vi "DigitalOutput-Drive.vi"(7 "duration (-1 = cont.)":i32=-1, 8 "error in":errorcluster, 9 "data":bool[](array[boolean]), 10 "line+TS":refnum<k21>, 11 "line only":refnum<k21>) -> (0 "error out":errorcluster)   [LabVIEW 2015]
doc: "Drives a DAQmx task [line only] to the level specified in the 1D Boolean array [data]. \n\nIf [duration] is nonnegative, then it will drive the task to ~[data] after the specified duration (ms). This is done using an asynchronous call to DigitalOutput-ScheduledDAQmxWrite.vi\n\nIf [line+TS] is a valid task (where a single timestamp line has been appended to the original task), then it will also pulse the timestamp line. The rising edge of this pulse is synchronized with the start of driving the line.\n\nIf [line+TS] is a valid task and [duration] is negative, then the [line only] task will never be driven. You can use this (with [data] as an empty array) to produce timestamp pulses.\n\nTiming warnings: The timestamp pulse is a 100-200 microsecond high pulse."
uses:
  <vilib>/DAQmx/write.llb/DAQmx Write (Digital 1D Bool NChan 1Samp 1Line).vi
  <vilib>/DAQmx/miscellaneous.llb/DAQmx Fill In Error Info.vi
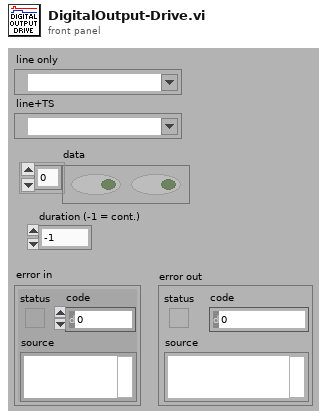
[diagram p1: front panel]
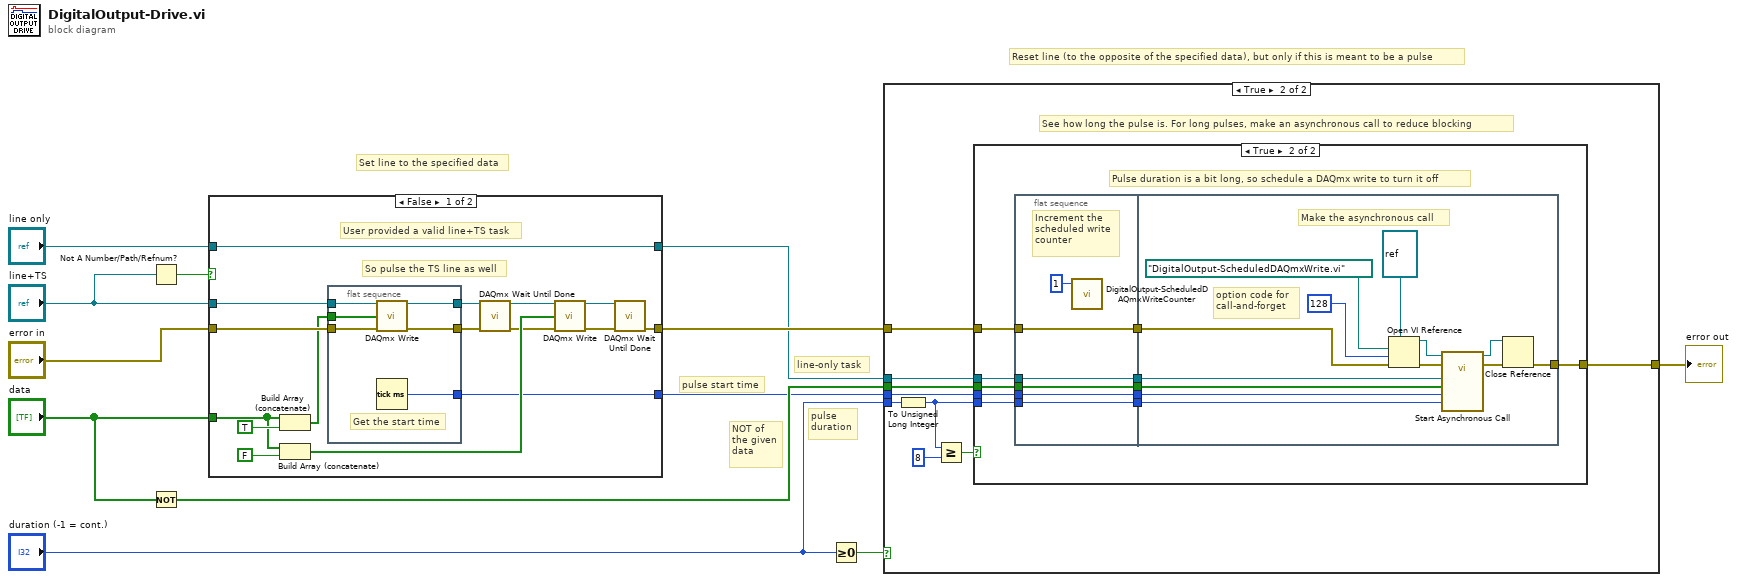
[diagram p0: block diagram]
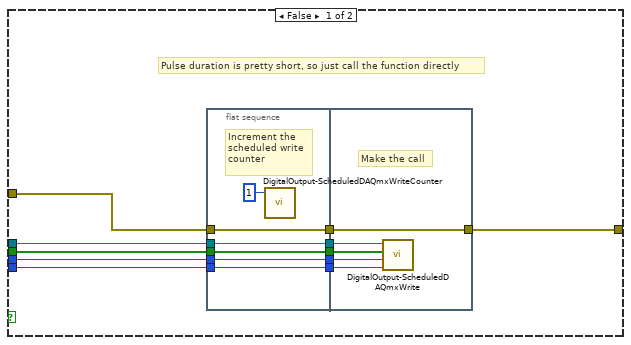
[diagram p3: hidden frame]
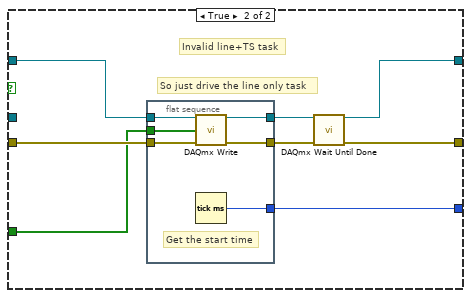
[diagram p4: hidden frame]
diagram:
  # "NOT of \nthe given\ndata"
  # "pulse\nduration"
  # "pulse start time"
  # "line-only task"
  # "Reset line (to the opposite of the specified data), but only if this is meant to be a pulse"
  # "Set line to the specified data"
  n1 = Not A Number/Path/Refnum?(number/path/refnum="line+TS") -> (NaN/Path/Refnum?=w12:bool)
  n2 = Not(x="data") -> (.not. x?=w6:bool[])
  n3 = case shown="False" w12 {
    tunnel: "line only" -> [w25 w42]
    tunnel: "line+TS" -> [w24 _]
    tunnel: "data" -> [w26 w36]
    tunnel: [w25 w39] -> w5
    tunnel: "error in" -> [w23 w37]
    tunnel: [w18 w38] -> w7
    tunnel: [w17 w35] -> w4
    frame False {
      # "User provided a valid line+TS task"
      # "So pulse the TS line as well"
      n4 = Build Array (concatenate)(w26, TRUE) -> (w22:bool[])
      n5 = Build Array (concatenate)(w26, FALSE) -> (w21:bool[])
      n6 = flat-sequence {
        tunnel: w24 -> [w34]
        tunnel: w23 -> [w33]
        tunnel: w22 -> [w32]
        tunnel: [w31] -> w16
        tunnel: [w30] -> w15
        tunnel: [w29] -> w17
        frame #0 {
          # "Get the start time"
          n7 = call-poly <vilib>:"DAQmx Write.vi"("task/channels in"=w34, "data"=w32, "error in"=w33) -> ("task out"=w31:refnum<k21>, "error out"=w30:errorcluster)  [unwired: 10 in, 1 out]
          n8 = Tick Count (ms)() -> (millisecond timer value=w29:u32)
        }
      }
      n9 = call <vilib>:"DAQmx Wait Until Done.vi"("task/channels in"=w16, "error in"=w15) -> ("task out"=w14:refnum<k21>, "error out"=w13:errorcluster)  [unwired: 12 in]
      n10 = call-poly <vilib>:"DAQmx Write.vi"("task/channels in"=w14, "data"=w21, "error in"=w13) -> ("task out"=w20:refnum<k21>, "error out"=w19:errorcluster)  [unwired: 10 in, 1 out]
      n11 = call <vilib>:"DAQmx Wait Until Done.vi"("task/channels in"=w20, "error in"=w19) -> ("error out"=w18:errorcluster)  [unwired: 12 in, 1 out]
    }
    frame True {
      # "So just drive the line only task"
      # "Invalid line+TS task"
      n12 = flat-sequence {
        tunnel: w42 -> [w48]
        tunnel: [w47] -> w41
        tunnel: [w46] -> w40
        tunnel: w37 -> [w45]
        tunnel: w36 -> [w44]
        tunnel: [w43] -> w35
        frame #0 {
          # "Get the start time"
          n13 = call-poly <vilib>:"DAQmx Write.vi"("task/channels in"=w48, "data"=w44, "error in"=w45) -> ("task out"=w47:refnum<k21>, "error out"=w46:errorcluster)  [unwired: 10 in, 1 out]
          n14 = Tick Count (ms)() -> (millisecond timer value=w43:u32)
        }
      }
      n15 = call <vilib>:"DAQmx Wait Until Done.vi"("task/channels in"=w41, "error in"=w40) -> ("task out"=w39:refnum<k21>, "error out"=w38:errorcluster)  [unwired: 12 in]
    }
  }
  n16 = Greater Or Equal To 0?(x="duration (-1 = cont.)") -> (x >= 0?=w2:bool)
  n17 = case shown="True" w2 {
    tunnel: w7 -> [w49 w58]
    tunnel: w6 -> [_ w57]
    tunnel: w5 -> [_ w56]
    tunnel: w4 -> [_ w55]
    tunnel: "duration (-1 = cont.)" -> [_ w54]
    tunnel: [w49 w53] -> w1
    frame False {
      # "Pulse duration negative, so this is supposed to be a\ncontinuous drive. So leave it as it is. Do nothing."
    }
    frame True {
      # "See how long the pulse is. For long pulses, make an asynchronous call to reduce blocking"
      n18 = To Unsigned Long Integer(number=w54) -> (unsigned 32bit integer=w52:u32)
      n19 = Greater Or Equal?(x=w52, y=u32 8) -> (x >= y?=w50:bool)
      n20 = case shown="True" w50 {
        tunnel: w58 -> [w64 w86]
        tunnel: w57 -> [w62 w85]
        tunnel: w56 -> [w63 w84]
        tunnel: w55 -> [w61 w83]
        tunnel: [w59 w82] -> w53
        tunnel: w52 -> [w60 w81]
        frame False {
          # "Pulse duration is pretty short, so just call the function directly"
          n21 = flat-sequence {
            tunnel: w60 -> [w71]
            tunnel: w61 -> [w72]
            tunnel: w63 -> [w73]
            tunnel: w62 -> [w74]
            tunnel: w64 -> [w75]
            tunnel: [w75] -> w69
            tunnel: [w74] -> w68
            tunnel: [w73] -> w67
            tunnel: [w72] -> w66
            tunnel: [w71] -> w65
            tunnel: w69 -> [w76]
            tunnel: w68 -> [w79]
            tunnel: w67 -> [w80]
            tunnel: w66 -> [w78]
            tunnel: w65 -> [w77]
            tunnel: [w76] -> w59
            frame #0 {
              # "Increment the\nscheduled write\ncounter"
              n22 = call "DigitalOutput-ScheduledDAQmxWriteCounter.vi"("Change in count"=i16 1) -> ()  [unwired: 3 in, 2 out]
            }
            frame #1 {
              # "Make the call"
              n23 = call "DigitalOutput-ScheduledDAQmxWrite.vi"("ms to wait"=w77, "Start time"=w78, "data"=w79, "task in"=w80) -> ()  [unwired: 1 in]
            }
          }
        }
        frame True {
          # "Pulse duration is a bit long, so schedule a DAQmx write to turn it off"
          n24 = flat-sequence {
            tunnel: w81 -> [w93]
            tunnel: w83 -> [w94]
            tunnel: w84 -> [w95]
            tunnel: w85 -> [w96]
            tunnel: w86 -> [w97]
            tunnel: [w97] -> w91
            tunnel: [w96] -> w90
            tunnel: [w95] -> w89
            tunnel: [w94] -> w88
            tunnel: [w93] -> w87
            tunnel: [w98] -> w82
            tunnel: w91 -> [w103]
            tunnel: w90 -> [w102]
            tunnel: w89 -> [w101]
            tunnel: w88 -> [w100]
            tunnel: w87 -> [w99]
            frame #0 {
              # "Increment the\nscheduled write\ncounter"
              n25 = call "DigitalOutput-ScheduledDAQmxWriteCounter.vi"("Change in count"=i16 1) -> ()  [unwired: 3 in, 2 out]
            }
            frame #1 {
              # "Make the asynchronous call"
              # "option code for\ncall-and-forget"
              n26 = Open VI Reference(type specifier VI Refnum (for type only)=refnum<vi> refnum, vi path=path "DigitalOutput-ScheduledDAQmxWrite.vi", options=128, error in (no error)=w103) -> (vi reference=w109:refnum<vi>, error out=w110:errorcluster)  [unwired: 2 in]
              n27 = call-by-ref "Start Asynchronous Call"(reference=w109, error in=w110, "ms to wait"=w99, "Start time"=w100, "data"=w102, "task in"=w101) -> (reference out=w107:refnum<vi>, error out=w108:errorcluster)  [unwired: 1 in]
              n28 = Close Reference(reference=w107, error in (no error)=w108) -> (error out=w98:errorcluster)
            }
          }
        }
      }
    }
  }
  "error out" <- w1
